vi "Auto_Path Tracking_Security_KBS_TCP.vi"() -> ()   [LabVIEW 2015]
uses:
  <vilib>/Instr/_visa.llb/VISA Configure Serial Port (Instr).vi
  <vilib>/Utility/file.llb/Read Delimited Spreadsheet (DBL).vi
panel:
  in  "M/A":bool=TRUE
  out "bytes written":i32
  out "Tracking_Error(m)":dbl
  in  "SAVE":bool
  out "save state":bool
  out "F9P GPS Data":T1
  out "LidarSteers":T2
  out "ROIs":cluster{bool[]}
  in  "?":enum32{"State", "ETC", "GPS&BATT", "TCP"}(tab)
  in  "stop":bool
  in  "file path (dialog if empty)":path caption="RDDF"
  out "XY Graph":T3(graph)
  in  "Refresh":bool
  in  "Serial Name":refnum<visa-resource-name>="COM1"
  out "ERP_Serial_DATA(RAW)":string
  in  "Vel":u8=4
  out "AEB":bool
  out "Index(near vehicle)":i32
  out "WP_no.":i32
  in  "TCP 수동":bool
  out "x_lat_path":dbl[](array[numeric])
  out "y_long_path":dbl[](array[numeric])
  out "vel. path":dbl[](array[numeric])
  out "Path_Vel_arr":dbl[](array[numeric])
  out "Path_long_arr":dbl[](array[numeric])
  out "Path_lat_arr":dbl[](array[numeric])
  out "ERP_Receive":T4
  out "Steer_CMD(Deg)":dbl
  out "CMD_2_ERP":T5
  in  "COM":refnum<visa-resource-name>="COM12"
  out "Heading_M":dbl
  out "Heading_T":dbl
  out "F9P_Data_GPGGA_Raw":string
  out "TM_Y(long)":dbl format="%-#_10g M"
  out "TM_X(lat)":dbl format="%-#_10g M"
  in  "COM 2":refnum<visa-resource-name>="COM6"
  out "Batt_Volt":dbl
  out "Charge":dbl
  out "Discharge":dbl
  out "SOC":u8
  in  "Speed_CMD":u16
  in  "Gear_CMD":u8
  in  "Steer_CMD":i16
  in  "Brake_CMD":u8
  out "TCP_Lat":u64
  out "TCP_Long":u64
  out "Brake":u8
  out "Go&Stop_feed":u8
  out "Go&Stop_CMD":u8
  out "E-Stop":u8
  out "Robot_State":u8
  out "Robot_Mode":u8
  out "KHP":dbl
  out "IMU_Output":T6
  out "GPS_KHP":u16
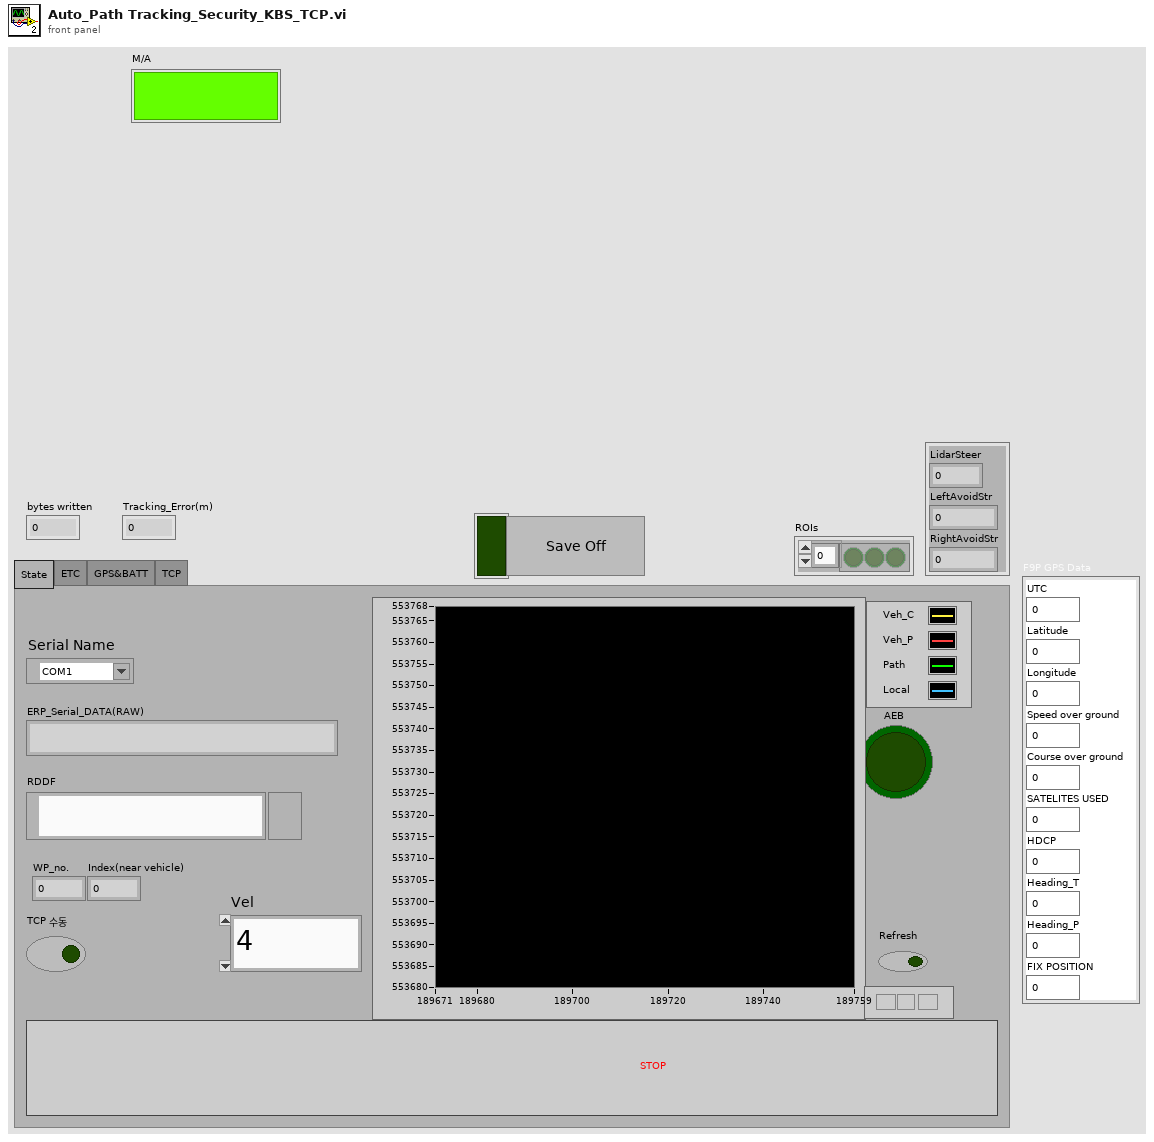
[diagram p1: front panel]
types:
  T1 = cluster{"UTC":dbl, "Latitude":dbl, "Longitude":dbl, "Speed over ground":dbl, "Course over ground":dbl, "SATELITES USED":i32, "HDCP":dbl, "Heading_T":dbl, "Heading_P":dbl, "FIX POSITION":i32}
  T2 = cluster{"LidarSteer":dbl, "LeftAvoidStr":dbl, "RightAvoidStr":dbl}
  T3 = cluster{"y_long_path":dbl[], "x_lat_path":dbl[]}[]
  T4 = cluster{"AorM":u8, "E-Stop":u8, "F_B":u8, "Speed":u16, "Steer":i16, "Brake":u8, "Encoder":u8, "Encoder 2":u8, "Encoder 3":u8, "Encoder 4":u8, "ALIVE":u8, "ETX_0":u8, "ETX_0 2":u8}
  T5 = cluster{"F/B":u8, "Speed":u16, "Steer":i16, "A/M":u8, "Brake":u8}
  T6 = cluster{"Acc_X":dbl, "Acc_Y":dbl, "Acc_Z":dbl, "Gyro_X":dbl, "Gyro_Y":dbl, "Gyro_Z":dbl, "Roll":dbl, "Pitch":dbl, "Yaw":dbl}
  T7 = cluster{"Robot_State_CMD":u8, "Robot_Mode_CMD":u8, "Path_Select":u8, "E-Stop":u8, "F_B":u8, "Speed":u16, "Steer":i16, "Brake":u8}
  T8 = cluster{"BATT_SOC":u8, "Robot_State":u8, "Robot_Mode":u8, "GPS_Lat":u32, "GPS_Long":u32, "Acc_X":i16, "Acc_Y":i16, "Acc_Z":i16, "Gyr_X":i16, "Gyr_Y":i16, "Gyr_Z":i16, "Ang_Roll":i16, "Ang_Pitch":i16, "Ang_Yaw":i16, "GPS_Speed":u16}
  T9 = cluster{"Packet_Size":u16, "Packet_Header":u16, "TCP_Lat":u32, "TCP_Long":u32, "Go&Stop_Feed":u8}
  T10 = enum16{"open", "replace", "create", "open or create", "replace or create", "replace or create with confirmation"}
  T11 = cluster{"S":u8, "T":u8, "X":u8, "AorM":u8, "E-Stop":u8, "F_B":u8, "Speed":u16, "Steer":i16, "Brake":u8, "ALIVE":u8, "ETX_0":u8, "ETX_0 2":u8}
  T12 = cluster{"Path_long_arr":dbl[], "Path_lat_arr":dbl[]}
  T13 = cluster{"Path_long_arr":dbl[], "Path_lat_arr":dbl[]}[]
  T14 = cluster{"UTC":dbl, "Latitude":dbl, "N/S":i8, "Longitude":dbl, "N/S":i8, "FIX POSITION":i32, "SATELITES USED":i32, "HDCP":dbl}
  T15 = cluster{"UTC":dbl, "N/S":i8, "Latitude":dbl, "N/S 2":i8, "Longitude":dbl, "N/S 3":i8, "Speed over ground":dbl, "Course over ground":dbl}
  T16 = cluster{"Heading_T":dbl, "T":i8, "Heading_M":dbl, "M":i8, "G_Speed_Knote":dbl, "N":i8, "G_Speed_KPH":dbl}
  T17 = enum16{"big-endian, network order", "native, host order", "little-endian"}
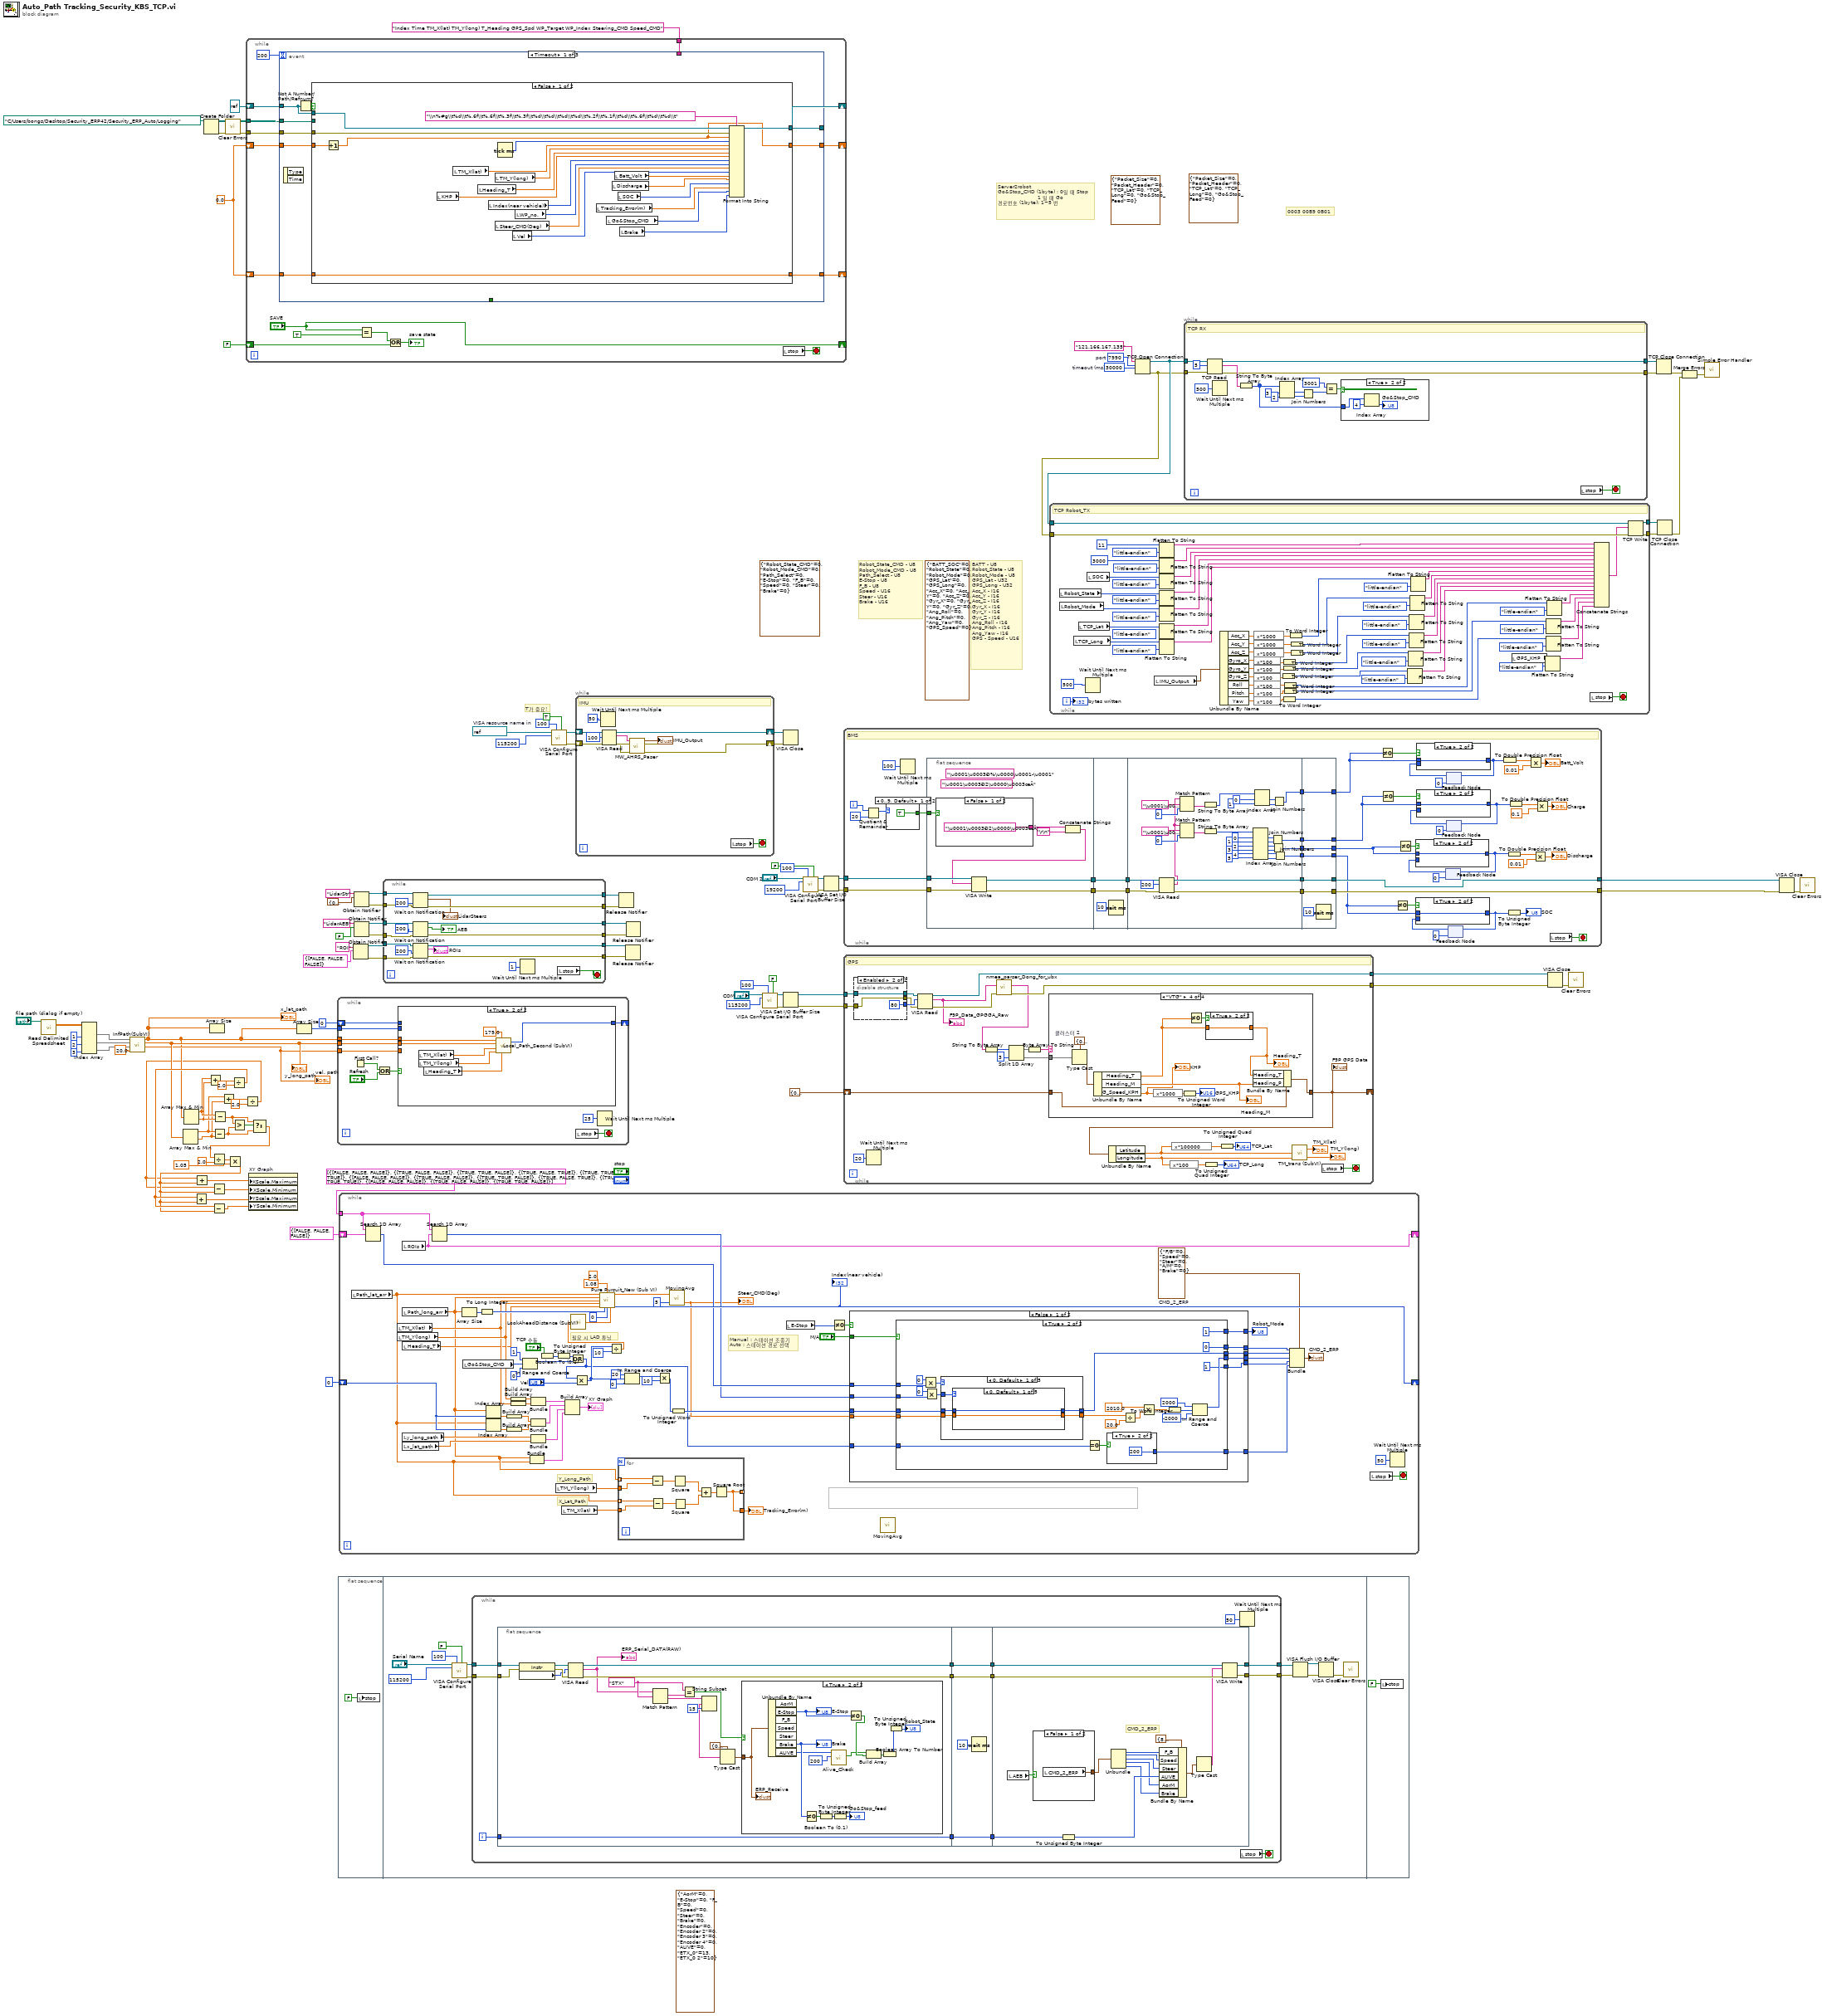
[diagram p0: block diagram]
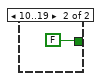
[diagram p7: hidden frame]
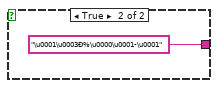
[diagram p8: hidden frame]
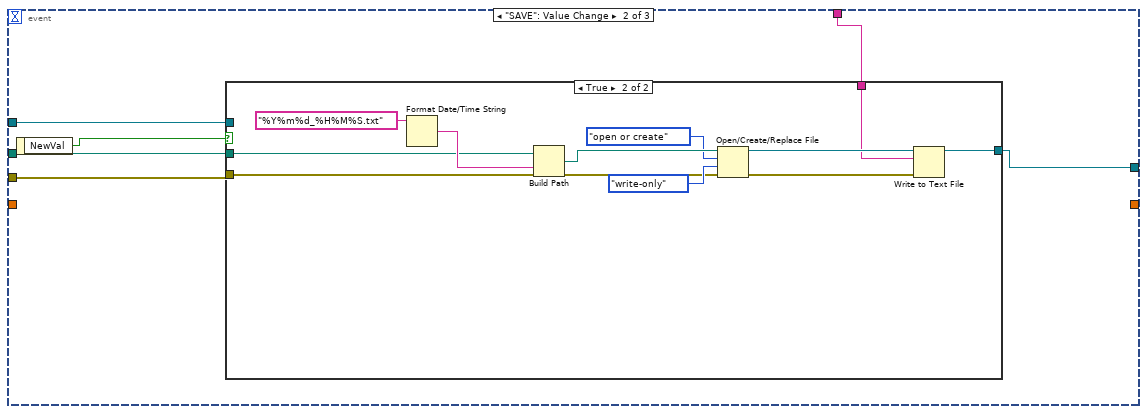
[diagram p10: hidden frame]
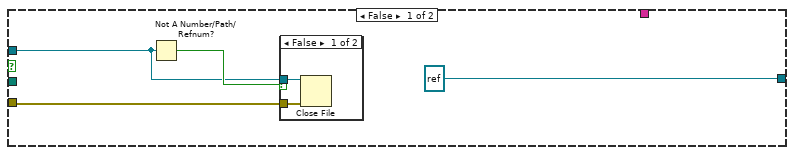
[diagram p11: hidden frame]
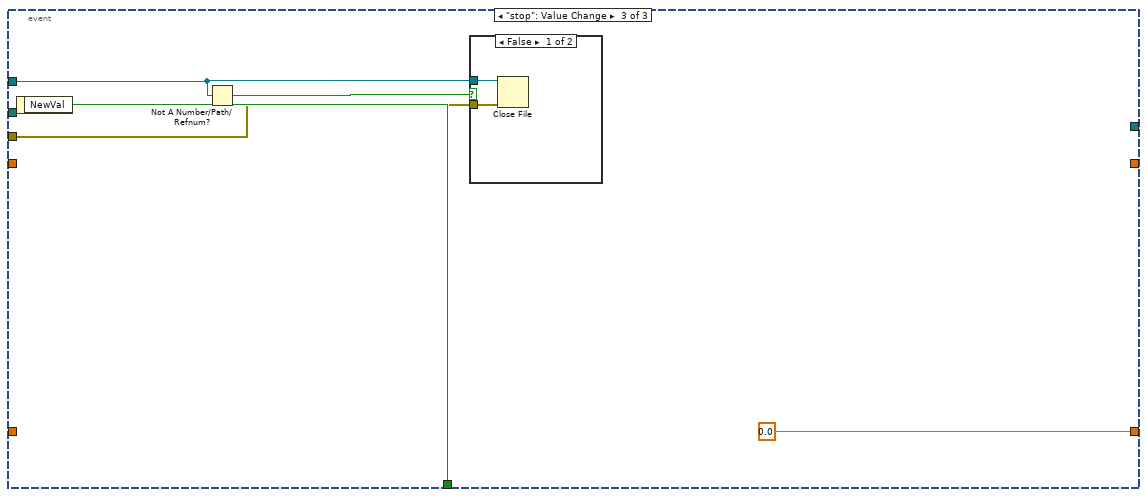
[diagram p13: hidden frame]
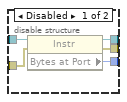
[diagram p15: hidden frame]
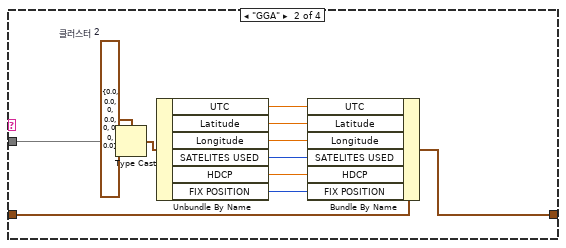
[diagram p17: hidden frame]
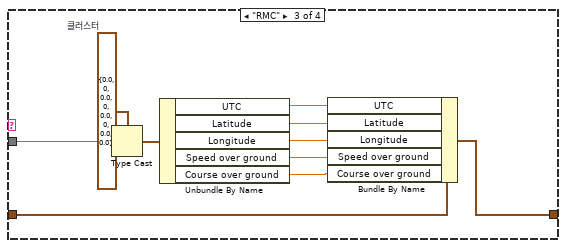
[diagram p18: hidden frame]
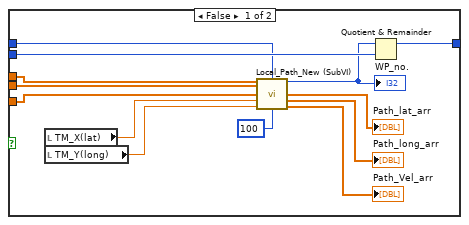
[diagram p20: hidden frame]
diagram:
  (unwired) T4 {"AorM"=0, "E-Stop"=0, "F_B"=0, "Speed"=0, "Steer"=0, "Brake"=0, "Encoder"=0, "Encoder 2"=0, "Encoder 3"=0, "Encoder 4"=0, "ALIVE"=0, "ETX_0"=13, "ETX_0 2"=10}
  (unwired) T7 {"Robot_State_CMD"=0, "Robot_Mode_CMD"=0, "Path_Select"=0, "E-Stop"=0, "F_B"=0, "Speed"=0, "Steer"=0, "Brake"=0} ("Server2Robot")
  (unwired) T8 {"BATT_SOC"=0, "Robot_State"=0, "Robot_Mode"=0, "GPS_Lat"=0, "GPS_Long"=0, "Acc_X"=0, "Acc_Y"=0, "Acc_Z"=0, "Gyr_X"=0, "Gyr_Y"=0, "Gyr_Z"=0, "Ang_Roll"=0, "Ang_Pitch"=0, "Ang_Yaw"=0, "GPS_Speed"=0} ("Robot2Server")
  w2 = u16 7990  # port
  w3 = 30000  # timeout (ms)
  w18 = refnum<visa-resource-name> "COM14"  # VISA resource name in
  (unwired) T9 {"Packet_Size"=0, "Packet_Header"=0, "TCP_Lat"=0, "TCP_Long"=0, "Go&Stop_Feed"=0}
  (unwired) T9 {"Packet_Size"=0, "Packet_Header"=0, "TCP_Lat"=0, "TCP_Long"=0, "Go&Stop_Feed"=0}
  w32 = 0.0 ("Distance(Encoder)")
  # "Robot_State_CMD - U8\nRobot_Mode_CMD - U8\nPath_Select - U8\nE-Stop - U8\nF_B - U8\nSpeed - U16\nSteer - U16\nBrake - U16"
  # "BATT - U8\nRobot_State - U8\nRobot_Mode - U8\nGPS_Lat - U32\nGPS_Long - U32\nAcc_X - I16\nAcc_Y - I16\nAcc_Z - I16\nGyr_X - I16\nGyr_Y - I16\nGyr_Z - I16\nAng_Roll - I16\nAng_Pitch - I16\nAng_Yaw - I16\nGPS - Speed - U16"
  # "T가 중요!"
  # "0003 00B9 0B01"
  # "Server2robot\nGo&Stop_CMD (1byte) : 0일 때 Stop\n                        1 일 때 Go\n경로번호 (1byte): 1~5 번"
  n1 = call-poly <vilib>:"Read Delimited Spreadsheet.vi"("file path (dialog if empty)"="file path (dialog if empty)") -> ("all rows"=w76:dbl[][])  [unwired: 9 in, 5 out]
  n2 = Index Array(array=w76, index (col) #1=1 ("비활성화된 인덱스 (열)"), index (col) #2=2 ("인덱스 (열)"), index (col) #3=3 ("인덱스 (열)")) -> (element #1=w105:dbl[], element #2=w104:dbl[], element #3=w103:dbl[])  [unwired: 3 in]
  n3 = call "InfPath(SubVI).vi"("Mod dist."=20.0, "vel."=w103, "y_long"=w104, "x_lat"=w105) -> ("vel. path"=w78:dbl[], "y_long_path"=w80:dbl[], "x_lat_path"=w77:dbl[])  [unwired: 1 out]
  "x_lat_path" <- w77
  "y_long_path" <- w80
  "vel. path" <- w78
  n4 = Array Max & Min(array=w80) -> (max value=w91:dbl, min value=w90:dbl)  [unwired: 2 out]
  n5 = Array Max & Min(array=w77) -> (max value=w97:dbl, min value=w96:dbl)  [unwired: 2 out]
  n6 = Create Folder(path (use dialog)=path "C:/Users/bongs/Desktop/Security_ERP42/Security_ERP_Auto/Logging") -> (created path=w35:path, error out=w33:errorcluster)  [unwired: 2 in, 1 out]
  n7 = Add(x=w97, y=w96) -> (x+y=w94:dbl)
  n8 = Array Size(array=w77) -> ()  [unwired: 1 out]
  n9 = Subtract(x=w91, y=w90) -> (x-y=w100:dbl)
  n10 = Subtract(x=w97, y=w96) -> (x-y=w101:dbl)
  n11 = Add(x=w91, y=w90) -> (x+y=w93:dbl)
  n12 = call <vilib>:"Clear Errors.vi"("error in (no error)"=w33) -> ("error out"=w34:errorcluster)  [unwired: 5 in, 1 out]
  n13 = Divide(x=w94, y=2.0) -> (x/y=w87:dbl)
  n14 = Greater?(x=w101, y=w100) -> (0:w102:bool)
  n15 = Divide(x=w93, y=2.0) -> (x/y=w74:dbl)
  n16 = while {
    tunnel: w34 -> [w123]
    tunnel: w35 -> [w122]
    shift-right: [w121] -> _
    shift-left: refnum<file> refnum ("refnum out") -> [w120]
    shift-right: [w119] -> _
    shift-left: w32 -> [w118]
    tunnel: "Index Time TM_X(lat) TM_Y(long) T_Heading GPS_Spd WP_Target WP_Index Steering_CMD Speed_CMD" ("포맷 문자열") -> [w117]
    shift-right: [w115] -> _
    shift-left: w32 -> [w116]
    shift-right: ["SAVE"] -> _
    shift-left: FALSE -> [w109]
    stop <- w110 stop-if-true
    n17 = event shown="[0] Timeout" {
      selector: _ -> [_ _ _]
      dyn-events: _ -> [_ _ _]
      timeout: 200 -> [_ _ _]
      tunnel: w123 -> [w131 w162 w183]
      tunnel: w122 -> [w132 w164 _]
      tunnel: [_ _ w186] -> _
      tunnel: [w129 w163 _] -> w121
      tunnel: w120 -> [w130 w160 w184]
      tunnel: [w127 _ 0.0 ("Distance(Encoder)")] -> w119
      tunnel: w118 -> [w128 _ _]
      tunnel: w117 -> [_ w159 _]
      tunnel: w116 -> [w126 _ _]
      tunnel: [w125 _ _] -> w115
      event Timeout {
        n18 = event-data() -> ()  [unwired: 1 in, 2 out]
        n19 = Not A Number/Path/Refnum?(number/path/refnum=w130) -> (NaN/Path/Refnum?=w133:bool)
        n20 = case shown="False" w133 {
          tunnel: w132 -> [_ _]
          tunnel: w131 -> [w155 _]
          tunnel: w130 -> [w154 w158]
          tunnel: [w153 w158] -> w129
          tunnel: w128 -> [w152 w157]
          tunnel: [w152 w157] -> w127
          tunnel: w126 -> [w151 w156]
          tunnel: [w149 w156] -> w125
          frame False {
            n21 = Increment(x=w151) -> (x+1=w149:dbl)
            n22 = local read "KHP"() -> (w144:dbl)
            n23 = local read "TM_X(lat)"() -> (w147:dbl)
            n24 = local read "Heading_T"() -> (w145:dbl)
            n25 = local read "Index(near vehicle)"() -> (w143:i32)
            n26 = local read "TM_Y(long)"() -> (w146:dbl)
            n27 = local read "Steer_CMD(Deg)"() -> (w141:dbl)
            n28 = Tick Count (ms)() -> (millisecond timer value=w148:u32)
            n29 = local read "Vel"() -> (w140:u8)
            n30 = local read "WP_no."() -> (w142:i32)
            n31 = local read "Tracking_Error(m)"() -> (w136:dbl)
            n32 = local read "Go&Stop_CMD"() -> (w135:u8)
            n33 = local read "Discharge"() -> (w138:dbl)
            n34 = local read "Batt_Volt"() -> (w139:dbl)
            n35 = local read "SOC"() -> (w137:u8)
            n36 = local read "Brake"() -> (w134:u8)
            n37 = Format Into String(format string="\\n%#g\\t%d\\t%.6f\\t%.6f\\t%.3f\\t%.3f\\t%d\\t%d\\t%d\\t%d\\t%.2f\\t%.1f\\t%d\\t%.6f\\t%d\\t%d\\t" ("포맷 문자열"), initial string=w154, error in=w155, w149, w148, w147, w146, w145, w144, w143, w142, w141, w140, w139, w138, w137, w136, w135, w134) -> (resulting string=w153:refnum<file>)  [unwired: 1 out]
          }
          frame True {
          }
        }
      }
      event "SAVE": Value Change {
        n38 = event-data() -> ("NewVal"=w161:bool)  [unwired: 1 in]
        n39 = case shown="True" w161 {
          tunnel: w164 -> [_ w179]
          tunnel: [refnum<file> refnum ("refnum out") w173] -> w163
          tunnel: w162 -> [w165 w175]
          tunnel: w160 -> [w167 _]
          tunnel: w159 -> [_ w172]
          frame False {
            n40 = Not A Number/Path/Refnum?(number/path/refnum=w167) -> (NaN/Path/Refnum?=w168:bool)
            n41 = case shown="False" w168 {
              tunnel: w167 -> [w170 _]
              tunnel: w165 -> [w169 _]
              frame False {
                n42 = Close File(refnum=w170, error in=w169) -> ()  [unwired: 2 out]
              }
              frame True {
              }
            }
          }
          frame True {
            n43 = Format Date/Time String(time format string (%c)="%Y%m%d_%H%M%S.txt" ("시간 포맷 문자열 (%c)")) -> (date/time string=w180:string)  [unwired: 2 in]
            n44 = Build Path(base path=w179, name or relative path=w180) -> (appended path=w178:path)
            n45 = Open/Create/Replace File(file path (use dialog)=w178, error in=w175, operation (0:open)=T10."open or create" ("동작(0:open)"), access (0:read/write)=enum16{"read/write", "read-only", "write-only"}."write-only" ("접근(0:읽기/쓰기)")) -> (refnum out=w174:refnum<file>, error out=w171:errorcluster)  [unwired: 2 in, 1 out]
            n46 = Write to Text File(file (use dialog)=w174, text=w172, error in=w171) -> (refnum out=w173:refnum<file>)  [unwired: 1 in, 2 out]
          }
        }
      }
      event "stop": Value Change {
        n47 = event-data() -> ("NewVal"=w186:bool)  [unwired: 1 in]
        n48 = Not A Number/Path/Refnum?(number/path/refnum=w184) -> (NaN/Path/Refnum?=w185:bool)
        n49 = case shown="False" w185 {
          tunnel: w184 -> [w188 _]
          tunnel: w183 -> [w187 _]
          frame False {
            n50 = Close File(refnum=w188, error in=w187) -> ()  [unwired: 2 out]
          }
          frame True {
          }
        }
      }
    }
    n51 = Equal?(x="SAVE", y=TRUE) -> (x = y?=w113:bool)
    n52 = Or(x=w113, y=w109) -> (x .or. y?=→"save state":bool)
    n53 = local read "stop"() -> (w110:bool)
  }
  n54 = Select(t=w101, s=w102, f=w100) -> (s? t:f=w98:dbl)
  n55 = Divide(x=w98, y=2.0) -> (x/y=w89:dbl)
  n56 = Multiply(x=w89, y=1.05) -> (x*y=w86:dbl)
  n57 = Add(x=w87, y=w86) -> (x+y=w84:dbl)
  n58 = Add(x=w74, y=w86) -> (x+y=w82:dbl)
  n59 = Subtract(x=w74, y=w86) -> (x-y=w83:dbl)
  n60 = Subtract(x=w87, y=w86) -> (x-y=w85:dbl)
  n61 = property on="XY Graph" class="XYGraph (strict)"("XScale.Maximum"=w82, "XScale.Minimum"=w83, "YScale.Maximum"=w84, "YScale.Minimum"=w85) -> ()  [unwired: 2 in, 2 out]
  n62 = Array Size(array=w77) -> (size(s)=w79:i32)
  n63 = while {
    tunnel: w77 -> [w198]
    tunnel: w80 -> [w197]
    tunnel: w78 -> [w195]
    tunnel: w79 -> [w194]
    shift-right: [w193] -> _
    shift-left: 0 ("Index0") -> [w196]
    stop <- w199 stop-if-true
    n64 = First Call?() -> (First Call?: T/F=w191:bool)
    n65 = Or(x=w191, y="Refresh") -> (x .or. y?=w192:bool)
    n66 = case shown="True" w192 {
      tunnel: w198 -> [w200 w219]
      tunnel: w197 -> [w202 w218]
      tunnel: w196 -> [w207 _]
      tunnel: w195 -> [w201 _]
      tunnel: w194 -> [w211 _]
      tunnel: [w212 w213] -> w193
      frame False {
        n67 = local read "TM_X(lat)"() -> (w210:dbl)
        n68 = local read "TM_Y(long)"() -> (w209:dbl)
        n69 = call "Local_Path_New (SubVI).vi"("x_lat_arr"=w200, "WP no_pre"=w207, "y_long_arr"=w202, "vel_arr"=w201, "x_lat_c"=w210, "y_long_c"=w209, "# of pnt"=100) -> ("INDEX(Near Point)"=w203:i32, "Lat(Local)"=→"Path_lat_arr":dbl[], "Long(Local)"=→"Path_long_arr":dbl[], "Vel(Local)"=→"Path_Vel_arr":dbl[])  [unwired: 5 in]
        "WP_no." <- w203
        n70 = Quotient & Remainder(x=w203, y=w211) -> (x-y*floor(x/y)=w212:i32)  [unwired: 1 out]
      }
      frame True {
        n71 = local read "TM_X(lat)"() -> (w217:dbl)
        n72 = local read "TM_Y(long)"() -> (w216:dbl)
        n73 = local read "Heading_T"() -> (w215:dbl)
        n74 = call "Local_Path_Second (SubVI).vi"("heading_deg"=w215, "heading_limit"=179.0, "y_long"=w216, "x_lat"=w217, "Y_long_path"=w218, "X_lat_path"=w219) -> ("Index(near vehicle)"=w213:i32)  [unwired: 1 out]
      }
    }
    n75 = local read "stop"() -> (w199:bool)
    n76 = Wait Until Next ms Multiple(millisecond multiple=u32 25) -> ()  [unwired: 1 out]
  }
  n77 = flat-sequence {
    frame #0 {
      n78 = local write "stop"(FALSE ("STop")) -> ()
    }
    frame #1 {
      n79 = call-poly "VISA Configure Serial Port"("VISA resource name"="Serial Name", "timeout (10sec)"=u32 100, "Enable Termination\nChar (T)"=FALSE ("Enable Termination\nChar (T)"), "baud rate (9600)"=u32 115200) -> ("VISA resource name out"=w223:refnum<visa-resource-name>, "error out"=w222:errorcluster)  [unwired: 10 in]
      n80 = while {
        tunnel: w223 -> [w243]
        tunnel: w222 -> [w242]
        tunnel: [w240] -> w225
        tunnel: [w239] -> w224
        i -> [w241]
        stop <- w232 stop-if-true
        n81 = flat-sequence {
          tunnel: w243 -> [w261]
          tunnel: w242 -> [w260]
          tunnel: [w259] -> w238
          tunnel: [w258] -> w236
          tunnel: w241 -> [w257]
          tunnel: [w257] -> w234
          tunnel: w238 -> [w278]
          tunnel: [w278] -> w237
          tunnel: w236 -> [w277]
          tunnel: [w277] -> w235
          tunnel: w234 -> [w276]
          tunnel: [w276] -> w233
          tunnel: w237 -> [w292]
          tunnel: w235 -> [w291]
          tunnel: w233 -> [w289]
          tunnel: [w288] -> w240
          tunnel: [w287] -> w239
          frame #0 {
            w251 = "STX" ("검색 문자열/문자 (-)")
            n82 = property class="Instr"(reference=w261, error in=w260) -> (reference out=w254:refnum<visa-resource-name>, error out=w256:errorcluster, "Serial Settings:Number of Bytes at Serial Port"=w255:u32)
            n83 = VISA Read(VISA resource name=w254, byte count=w255, error in (no error)=w256) -> (VISA resource name out=w259:refnum<visa-resource-name>, read buffer=w249:string, error out=w258:errorcluster)  [unwired: 1 out]
            "ERP_Serial_DATA(RAW)" <- w249
            n84 = Match Pattern(string=w249, regular expression=w251) -> (match substring=w250:string, after substring=w253:string)  [unwired: 1 in, 2 out]
            n85 = Equal?(x=w251, y=w250) -> (x = y?=w248:bool)
            n86 = String Subset(string=w253, length (rest)=15 ("길이(나머지)")) -> (substring=w247:string)  [unwired: 1 in]
            n87 = Type Cast(type=T4 {"AorM"=0, "E-Stop"=0, "F_B"=0, "Speed"=0, "Steer"=0, "Brake"=0, "Encoder"=0, "Encoder 2"=0, "Encoder 3"=0, "Encoder 4"=0, "ALIVE"=0, "ETX_0"=13, "ETX_0 2"=10}, x=w247) -> (*(type *) &x=w245:T4)
            n88 = case shown="True" w248 {
              tunnel: w245 -> [_ w270]
              frame False {
              }
              frame True {
                n89 = Unbundle By Name(w270) -> ("E-Stop"=w267:u8, "Brake"=w274:u8, "ALIVE"=w269:u8)  [unwired: 4 out]
                "Brake" <- w274
                "E-Stop" <- w267
                n90 = Not Equal To 0?(x=w274) -> (x != 0?=w273:bool)
                n91 = Boolean To (0,1)(Boolean=w273) -> (0, 1=w272:i16)
                n92 = call "Alive_Check.vi"("Timeout_msec"=u32 200, "Alv_cnt"=w269) -> ("Timeout"=w262:bool)  [unwired: 8 in, 1 out]
                n93 = To Unsigned Byte Integer(number=w272) -> (unsigned 8bit integer=→"Go&Stop_feed":u8)
                n94 = Not Equal To 0?(x=w267) -> (x != 0?=w263:bool)
                n95 = Build Array(w262, w263) -> (w266:bool[])
                n96 = Boolean Array To Number(Boolean array=w266) -> (number=w265:u32)
                n97 = To Unsigned Byte Integer(number=w265) -> (unsigned 8bit integer=→"Robot_State":u8)
                "ERP_Receive" <- w270
              }
            }
          }
          frame #1 {
            n98 = Wait (ms)(milliseconds to wait=u32 10 ("대기 시간(ms)")) -> ()  [unwired: 1 out]
          }
          frame #2 {
            # "CMD_2_ERP"
            n99 = local read "AEB"() -> (w280:bool)
            n100 = case shown="False" w280 {
              tunnel: [w295 w296] -> w281
              frame False {
                n101 = local read "CMD_2_ERP"() -> (w295:T5)
              }
              frame True {
                w296 = T5 {"F/B"=0, "Speed"=0, "Steer"=0, "A/M"=1, "Brake"=200}  # CMD_2_ERP
              }
            }
            n102 = To Unsigned Byte Integer(number=w289) -> (unsigned 8bit integer=w294:u8)
            n103 = Unbundle(w281) -> ("F/B"=w286:u8, "Speed"=w285:u16, "Steer"=w284:i16, "A/M"=w282:u8, "Brake"=w279:u8)
            n104 = Bundle By Name(cluster=T11 {"S"=83, "T"=84, "X"=88, "AorM"=0, "E-Stop"=0, "F_B"=0, "Speed"=0, "Steer"=0, "Brake"=0, "ALIVE"=0, "ETX_0"=13, "ETX_0 2"=10}, "F_B"=w286, "Speed"=w285, "Steer"=w284, "ALIVE"=w294, "AorM"=w282, "Brake"=w279) -> (w293:T11)
            n105 = Type Cast(x=w293) -> (*(type *) &x=w290:string)  [unwired: 1 in]
            n106 = VISA Write(VISA resource name=w292, write buffer=w290, error in (no error)=w291) -> (VISA resource name out=w288:refnum<visa-resource-name>, error out=w287:errorcluster)  [unwired: 1 out]
          }
        }
        n107 = Wait Until Next ms Multiple(millisecond multiple=u32 50 ("ms 배수")) -> ()  [unwired: 1 out]
        n108 = local read "stop"() -> (w232:bool)
      }
      n109 = VISA Flush I/O Buffer(VISA resource name=w225, error in (no error)=w224) -> (VISA resource name out=w226:refnum<visa-resource-name>, error out=w227:errorcluster)  [unwired: 1 in]
      n110 = VISA Close(VISA resource name=w226, error in (no error)=w227) -> (error out=w221:errorcluster)
      n111 = call <vilib>:"Clear Errors.vi"("error in (no error)"=w221) -> ()  [unwired: 5 in, 2 out]
    }
    frame #2 {
      n112 = local write "stop"(FALSE ("STop")) -> ()
    }
  }
  n113 = while {
    shift-right: [w351] -> _
    shift-left: 0 -> [w346]
    shift-right: [w330] -> _
    shift-left: cluster{bool[]} {[FALSE, FALSE, FALSE]} -> [w333]
    tunnel: cluster{bool[]}[] [{[FALSE, FALSE, FALSE]}, {[TRUE, FALSE, FALSE]}, {[TRUE, TRUE, FALSE]}, {[TRUE, FALSE, TRUE]}, {[TRUE, TRUE, TRUE]}, {[FALSE, FALSE, FALSE]}, {[TRUE, FALSE, FALSE]}, {[TRUE, TRUE, FALSE]}, {[TRUE, FALSE, TRUE]}, {[TRUE, TRUE, TRUE]}, {[FALSE, FALSE, FALSE]}, {[TRUE, FALSE, FALSE]}, {[TRUE, TRUE, FALSE]}] -> [w334]
    stop <- w355 stop-if-true
    w317 = T5 {"F/B"=0, "Speed"=0, "Steer"=0, "A/M"=0, "Brake"=0}  # CMD_2_ERP
    (unwired) 2.0 ("L")
    # "Manual : 스테이션 조종기\nAuto : 스테이션 경로 선택"
    # "X_Lat_Path"
    # "Y_Long_Path"
    # "필요 시 LAD 튜닝"
    n114 = local read "Path_lat_arr"() -> (w309:dbl[])
    n115 = Search 1D Array(1D array=w334, element=w333) -> (index of element=w332:i32)  [unwired: 1 in]
    n116 = local read "TM_X(lat)"() -> (w347:dbl)
    n117 = local read "TM_Y(long)"() -> (w348:dbl)
    n118 = local read "y_long_path"() -> (w323:dbl[])
    n119 = local read "x_lat_path"() -> (w322:dbl[])
    n120 = local read "ROIs"() -> (w330:cluster{bool[]})
    n121 = local read "Path_long_arr"() -> (w310:dbl[])
    n122 = local read "Heading_T"() -> (w342:dbl)
    n123 = Search 1D Array(1D array=w334, element=w330) -> (index of element=w331:i32)  [unwired: 1 in]
    n124 = Array Size(array=w310) -> (size(s)=w352:i32)
    n125 = local read "Go&Stop_CMD"() -> (w311:u8)
    n126 = To Long Integer(number=w352) -> (32bit integer=w350:i32)
    n127 = Index Array(array=w310, index=w346) -> (element=w359:dbl)
    n128 = Index Array(array=w309, index=w346) -> (element=w358:dbl)
    n129 = Build Array(w359) -> (w357:dbl[])
    n130 = Build Array(w358) -> (w356:dbl[])
    n131 = Build Array(w348) -> (w361:dbl[])
    n132 = Build Array(w347) -> (w360:dbl[])
    n133 = In Range and Coerce(upper limit=u8 1, x=w311, lower limit=u8 0) -> (coerced(x)=w308:u8)  [unwired: 1 out]
    n134 = Bundle("Path_long_arr"=w310, "Path_lat_arr"=w309) -> (w338:T12)  [unwired: 1 in]
    n135 = Bundle(w361, w360) -> (w344:cluster{dbl[], dbl[]})  [unwired: 1 in]
    n136 = Bundle(w357, w356) -> (w343:cluster{dbl[], dbl[]})  [unwired: 1 in]
    n137 = Bundle("y_long_path"=w323, "x_lat_path"=w322) -> (w345:cluster{"y_long_path":dbl[], "x_lat_path":dbl[]})  [unwired: 1 in]
    n138 = Boolean To (0,1)(Boolean="TCP 수동") -> (0, 1=w307:i16)
    n139 = local read "TM_Y(long)"() -> (w320:dbl)
    n140 = To Unsigned Byte Integer(number=w307) -> (unsigned 8bit integer=w305:u8)
    n141 = local read "TM_X(lat)"() -> (w321:dbl)
    n142 = Build Array(w344, w343, w345, w338) -> (→"XY Graph":T13)
    n143 = Or(x=w305, y=w308) -> (x .or. y?=w304:u8)
    n144 = Multiply(x=w304, y="Vel") -> (x*y=w312:u8)
    n145 = Divide(x=w312, y=u8 10) -> (x/y=w339:dbl)
    n146 = call "LookAheadDistance (SubVI).vi"("velocity(kph)"=w339) -> ("ld(m)"=w341:dbl)
    n147 = call "Pure Pursuit_New (Sub VI).vi"("x_lat_path"=w309, "L"=1.08, "y_long_path"=w310, "X_Current"=w347, "Y_Current"=w348, "Heading_Current"=w342, "#pnt"=w350, "WP no_pre"=0, "LAD"=w341) -> ("Steer_CMD(Deg)"=w302:dbl, "Index(near vehicle)"=w351:i32)  [unwired: 5 in]
    "Index(near vehicle)" <- w351
    n148 = for {
      tunnel: w310 -> [w374] mode=indexing
      tunnel: w309 -> [w372] mode=indexing
      tunnel: w321 -> [w371]
      tunnel: w320 -> [w373]
      tunnel: [w365] -> _ mode=indexing
      tunnel: [w365] -> w319
      n149 = Subtract(x=w374, y=w373) -> (x-y=w370:dbl)
      n150 = Subtract(x=w372, y=w371) -> (x-y=w369:dbl)
      n151 = Square(x=w370) -> (x^2=w368:dbl)
      n152 = Square(x=w369) -> (x^2=w367:dbl)
      n153 = Add(x=w368, y=w367) -> (x+y=w366:dbl)
      n154 = Square Root(x=w366) -> (sqrt(x)=w365:dbl)
    }
    "Tracking_Error(m)" <- w319
    n155 = In Range and Coerce(upper limit=u8 20 ("상위 리미트"), x=w312, lower limit=u8 0 ("하위 리미트")) -> (coerced(x)=w327:u8)  [unwired: 1 out]
    n156 = Multiply(x=w327, y=u8 10) -> (x*y=w325:u8)
    n157 = call "MovingAvg.vi"("입력"=w302, "이동평균을 구할 자료의 개수"=u16 5) -> ("이동평균"=w301:dbl)  [unwired: 2 out]
    "Steer_CMD(Deg)" <- w301
    n158 = To Unsigned Word Integer(number=w325) -> (unsigned 16bit integer=w336:u16)
    n159 = local read "E-Stop"() -> (w299:u8)
    n160 = Not Equal To 0?(x=w299) -> (x != 0?=w335:bool)
    n161 = case shown="False" w335 {
      tunnel: [w378 w518] -> w364
      tunnel: [w384 w518] -> w363
      tunnel: [w383 w518] -> w362
      tunnel: [w377 w518] -> w337
      tunnel: w332 -> [w382 _]
      tunnel: w331 -> [w381 _]
      tunnel: w301 -> [w386 _]
      tunnel: w336 -> [w385 _]
      tunnel: [w380 u8 200] -> w318
      tunnel: w304 -> [w379 _]
      tunnel: "M/A" -> [w376 _]
      tunnel: [w375 w518] -> w298
      frame False {
        n162 = case shown="True" w376 {
          tunnel: w386 -> [_ w425]
          tunnel: w385 -> [_ w424]
          tunnel: [w397 w423] -> w384
          tunnel: [w392 w414] -> w383
          tunnel: w382 -> [_ w413]
          tunnel: w381 -> [_ w409]
          tunnel: [w387 w407] -> w380
          tunnel: w379 -> [_ w406]
          tunnel: ["Gear_CMD" u8 0] -> w378
          tunnel: [u8 1 u8 1] -> w377
          tunnel: [u8 0 u8 1] -> w375
          frame False {
            n163 = In Range and Coerce(upper limit=i16 2000, x="Steer_CMD", lower limit=i16 -2000) -> (coerced(x)=w392:i16)  [unwired: 1 out]
            n164 = In Range and Coerce(upper limit=u16 10, x="Speed_CMD", lower limit=u16 0) -> (coerced(x)=w397:u16)  [unwired: 1 out]
            n165 = In Range and Coerce(upper limit=u8 200, x="Brake_CMD", lower limit=u8 0) -> (coerced(x)=w387:u8)  [unwired: 1 out]
          }
          frame True {
            n166 = Multiply(x=0, y=w413) -> (x*y=w411:i32)
            n167 = Multiply(x=0, y=w409) -> (x*y=w408:i32)
            n168 = case shown="0, Default" w411 {
              tunnel: w425 -> [w430 w448 w466 w484 w502]
              tunnel: [w431 w449 w467 w485 w503] -> w415
              tunnel: w408 -> [w432 w450 w468 w486 w504]
              tunnel: [w429 w447 w465 w483 w501] -> w423
              tunnel: w424 -> [w428 w446 w464 w482 w500]
              frame 0, Default {
                n169 = case shown="0, Default" w432 {
                  tunnel: [w434 w436 w438 w441 w444] -> w431
                  tunnel: w430 -> [w434 w436 _ _ _]
                  tunnel: [w433 w435 w437 w440 w443] -> w429
                  tunnel: w428 -> [w433 w435 w437 w440 w443]
                  frame 0, Default {
                  }
                  frame 1 {
                  }
                  frame 2 {
                    n170 = local read "LidarSteers"() -> (w439:T2)
                    n171 = Unbundle By Name(w439) -> ("LeftAvoidStr"=w438:dbl)
                  }
                  frame 3 {
                    n172 = local read "LidarSteers"() -> (w442:T2)
                    n173 = Unbundle By Name(w442) -> ("RightAvoidStr"=w441:dbl)
                  }
                  frame 4 {
                    n174 = local read "LidarSteers"() -> (w445:T2)
                    n175 = Unbundle By Name(w445) -> ("LidarSteer"=w444:dbl)
                  }
                }
              }
              frame 1 {
                n176 = case shown="0, Default" w450 {
                  tunnel: [w452 w454 w456 w459 w462] -> w449
                  tunnel: w448 -> [w452 w454 _ _ _]
                  tunnel: [w451 w453 w455 w458 w461] -> w447
                  tunnel: w446 -> [w451 w453 w455 w458 w461]
                  frame 0, Default {
                  }
                  frame 1 {
                  }
                  frame 2 {
                    n177 = local read "LidarSteers"() -> (w457:T2)
                    n178 = Unbundle By Name(w457) -> ("LeftAvoidStr"=w456:dbl)
                  }
                  frame 3 {
                    n179 = local read "LidarSteers"() -> (w460:T2)
                    n180 = Unbundle By Name(w460) -> ("RightAvoidStr"=w459:dbl)
                  }
                  frame 4 {
                    n181 = local read "LidarSteers"() -> (w463:T2)
                    n182 = Unbundle By Name(w463) -> ("LidarSteer"=w462:dbl)
                  }
                }
              }
              frame 2 {
                n183 = case shown="1" w468 {
                  tunnel: [w470 w472 w474 w477 w480] -> w467
                  tunnel: w466 -> [w470 w472 _ _ _]
                  tunnel: [w469 w471 w473 w476 w479] -> w465
                  tunnel: w464 -> [w469 w471 w473 w476 w479]
                  frame 0, Default {
                  }
                  frame 1 {
                  }
                  frame 2 {
                    n184 = local read "LidarSteers"() -> (w475:T2)
                    n185 = Unbundle By Name(w475) -> ("LeftAvoidStr"=w474:dbl)
                  }
                  frame 3 {
                    n186 = local read "LidarSteers"() -> (w478:T2)
                    n187 = Unbundle By Name(w478) -> ("RightAvoidStr"=w477:dbl)
                  }
                  frame 4 {
                    n188 = local read "LidarSteers"() -> (w481:T2)
                    n189 = Unbundle By Name(w481) -> ("LidarSteer"=w480:dbl)
                  }
                }
              }
              frame 3 {
                n190 = case shown="0, Default" w486 {
                  tunnel: [w488 w490 w492 w495 w498] -> w485
                  tunnel: w484 -> [w488 w490 _ _ _]
                  tunnel: [w487 w489 w491 w494 w497] -> w483
                  tunnel: w482 -> [w487 w489 w491 w494 w497]
                  frame 0, Default {
                  }
                  frame 1 {
                  }
                  frame 2 {
                    n191 = local read "LidarSteers"() -> (w493:T2)
                    n192 = Unbundle By Name(w493) -> ("LeftAvoidStr"=w492:dbl)
                  }
                  frame 3 {
                    n193 = local read "LidarSteers"() -> (w496:T2)
                    n194 = Unbundle By Name(w496) -> ("RightAvoidStr"=w495:dbl)
                  }
                  frame 4 {
                    n195 = local read "LidarSteers"() -> (w499:T2)
                    n196 = Unbundle By Name(w499) -> ("LidarSteer"=w498:dbl)
                  }
                }
              }
              frame 4 {
                n197 = case shown="0, Default" w504 {
                  tunnel: [w506 w508 w510 w513 w516] -> w503
                  tunnel: w502 -> [w506 w508 _ _ _]
                  tunnel: [w505 w507 w509 w512 w515] -> w501
                  tunnel: w500 -> [w505 w507 w509 w512 w515]
                  frame 0, Default {
                  }
                  frame 1 {
                  }
                  frame 2 {
                    n198 = local read "LidarSteers"() -> (w511:T2)
                    n199 = Unbundle By Name(w511) -> ("LeftAvoidStr"=w510:dbl)
                  }
                  frame 3 {
                    n200 = local read "LidarSteers"() -> (w514:T2)
                    n201 = Unbundle By Name(w514) -> ("RightAvoidStr"=w513:dbl)
                  }
                  frame 4 {
                    n202 = local read "LidarSteers"() -> (w517:T2)
                    n203 = Unbundle By Name(w517) -> ("LidarSteer"=w516:dbl)
                  }
                }
              }
            }
            n204 = Equal To 0?(x=w406) -> (x = 0?=w405:bool)
            n205 = case shown="True" w405 {
              tunnel: [u8 0 u8 200] -> w407
              frame False {
              }
              frame True {
              }
            }
            n206 = Divide(x=w415, y=20.0) -> (x/y=w421:dbl)
            n207 = Multiply(x=2010.0, y=w421) -> (x*y=w420:dbl)
            n208 = To Word Integer(number=w420) -> (16bit integer=w422:i16)
            n209 = In Range and Coerce(upper limit=i16 2000 ("상위 리미트"), x=w422, lower limit=i16 -2000 ("하위 리미트")) -> (coerced(x)=w414:i16)  [unwired: 1 out]
          }
        }
      }
      frame True {
        w518 = u8 0
      }
    }
    "Robot_Mode" <- w298
    n210 = call "MovingAvg.vi"() -> ()  [unwired: 2 in, 3 out]
    n211 = Bundle(cluster=w317, "F/B"=w364, "Speed"=w363, "Steer"=w362, "A/M"=w337, "Brake"=w318) -> (→"CMD_2_ERP":T5)
    n212 = local read "stop"() -> (w355:bool)
    n213 = Wait Until Next ms Multiple(millisecond multiple=u32 50 ("ms 배수")) -> ()  [unwired: 1 out]
  }
  n214 = Obtain Notifier(name (unnamed)="ROI" ("이름(이름없음)"), notification data type=cluster{bool[]} {[FALSE, FALSE, FALSE]}) -> (notifier out=w58:refnum<notifier>, error out=w57:errorcluster)  [unwired: 2 in, 1 out]
  n215 = Obtain Notifier(name (unnamed)="LidarStr" ("이름(이름없음)"), notification data type=T2 {"LidarSteer"=0.0, "LeftAvoidStr"=0.0, "RightAvoidStr"=0.0}) -> (notifier out=w71:refnum<notifier>, error out=w69:errorcluster)  [unwired: 2 in, 1 out]
  n216 = Obtain Notifier(name (unnamed)="LidarAEB" ("이름(이름없음)"), notification data type=FALSE) -> (notifier out=w65:refnum<notifier>, error out=w62:errorcluster)  [unwired: 2 in, 1 out]
  n217 = while {
    tunnel: w71 -> [w537]
    tunnel: [w536] -> w70
    tunnel: w69 -> [w535]
    tunnel: [w534] -> w68
    tunnel: w65 -> [w533]
    tunnel: [w532] -> w64
    tunnel: w62 -> [w531]
    tunnel: [w529] -> w61
    tunnel: w58 -> [w526]
    tunnel: w57 -> [w525]
    tunnel: [w523] -> w56
    tunnel: [w522] -> w55
    stop <- w539 stop-if-true
    n218 = Wait on Notification(notifier=w537, timeout in ms (-1)=200 ("타임아웃(ms) (-1)"), error in (no error)=w535) -> (notifier out=w536:refnum<notifier>, notification=→"LidarSteers":T2, error out=w534:errorcluster)  [unwired: 1 in, 1 out]
    n219 = Wait on Notification(notifier=w533, timeout in ms (-1)=200 ("타임아웃(ms) (-1)"), error in (no error)=w531) -> (notifier out=w532:refnum<notifier>, notification=→"AEB":bool, error out=w529:errorcluster)  [unwired: 1 in, 1 out]
    n220 = Wait on Notification(notifier=w526, timeout in ms (-1)=200 ("타임아웃(ms) (-1)"), error in (no error)=w525) -> (notifier out=w523:refnum<notifier>, notification=→"ROIs":cluster{bool[]}, error out=w522:errorcluster)  [unwired: 1 in, 1 out]
    n221 = Wait Until Next ms Multiple(millisecond multiple=u32 1) -> ()  [unwired: 1 out]
    n222 = local read "stop"() -> (w539:bool)
  }
  n223 = call-poly "VISA Configure Serial Port"("VISA resource name"=w18, "timeout (10sec)"=u32 100, "Enable Termination\nChar (T)"=TRUE, "baud rate (9600)"=u32 115200) -> ("VISA resource name out"=w17:refnum<visa-resource-name>, "error out"=w16:errorcluster)  [unwired: 10 in]
  n224 = while {
    shift-right: [w549] -> w13
    shift-left: w17 -> [w545]
    shift-right: [w542] -> w12
    shift-left: w16 -> [w544]
    stop <- w541 stop-if-true
    # "IMU"
    n225 = Wait Until Next ms Multiple(millisecond multiple=u32 50) -> ()  [unwired: 1 out]
    n226 = VISA Read(VISA resource name=w545, byte count=u32 100, error in (no error)=w544) -> (VISA resource name out=w549:refnum<visa-resource-name>, read buffer=w547:string, error out=w548:errorcluster)  [unwired: 1 out]
    n227 = call "MW_AHRS_Paser.vi"("error"=w548, "String In"=w547) -> ("error IO"=w542:errorcluster, "Output"=→"IMU_Output":T6)  [unwired: 4 in]
    n228 = local read "stop"() -> (w541:bool)
  }
  n229 = Release Notifier(notifier=w70, error in (no error)=w68) -> ()  [unwired: 1 in, 3 out]
  n230 = Release Notifier(notifier=w56, error in (no error)=w55) -> ()  [unwired: 1 in, 3 out]
  n231 = Release Notifier(notifier=w64, error in (no error)=w61) -> ()  [unwired: 1 in, 3 out]
  n232 = call-poly "VISA Configure Serial Port"("VISA resource name"="COM", "timeout (10sec)"=u32 100, "Enable Termination\nChar (T)"=FALSE ("Enable Termination\nChar (T)"), "baud rate (9600)"=u32 115200 ("baud rate")) -> ("VISA resource name out"=w48:refnum<visa-resource-name>, "error out"=w47:errorcluster)  [unwired: 10 in]
  n233 = VISA Close(VISA resource name=w13, error in (no error)=w12) -> ()  [unwired: 1 out]
  n234 = VISA Set I/O Buffer Size(VISA resource name=w48, error in (no error)=w47) -> (VISA resource name out=w43:refnum<visa-resource-name>, error out=w42:errorcluster)  [unwired: 2 in]
  n235 = call-poly "VISA Configure Serial Port"("VISA resource name"="COM 2", "timeout (10sec)"=u32 100, "Enable Termination\nChar (T)"=FALSE ("Enable Termination\nChar (T)"), "baud rate (9600)"=u32 19200 ("baud rate")) -> ("VISA resource name out"=w28:refnum<visa-resource-name>, "error out"=w27:errorcluster)  [unwired: 10 in]
  n236 = VISA Set I/O Buffer Size(VISA resource name=w28, error in (no error)=w27) -> (VISA resource name out=w24:refnum<visa-resource-name>, error out=w23:errorcluster)  [unwired: 2 in]
  n237 = while {
    shift-right: [w568] -> _
    shift-left: T1 {"UTC"=0.0, "Latitude"=0.0, "Longitude"=0.0, "Speed over ground"=0.0, "Course over ground"=0.0, "SATELITES USED"=0, "HDCP"=0.0, "Heading_T"=0.0, "Heading_P"=0.0, "FIX POSITION"=0} ("Garmin GPS Data") -> [w576]
    tunnel: w43 -> [w560]
    tunnel: w42 -> [w558]
    tunnel: [w569] -> w46
    tunnel: [w575] -> w45
    stop <- w555 stop-if-true
    # "GPS"
    n238 = disable-structure shown="Enabled" {
      disable-tunnel: [w581 u32 80 ("Bytes at Port")] -> w561
      disable-tunnel: w560 -> [w580 w583]
      disable-tunnel: [w579 w583] -> w559
      disable-tunnel: w558 -> [w578 w582]
      disable-tunnel: [w577 w582] -> w557
      frame Disabled {
        n239 = property class="Instr"(reference=w580, error in=w578) -> (reference out=w579:refnum<visa-resource-name>, error out=w577:errorcluster, "Bytes at Port"=w581:u32)
      }
      frame Enabled {
      }
    }
    n240 = Wait Until Next ms Multiple(millisecond multiple=u32 20 ("타임아웃(ms) (-1)")) -> ()  [unwired: 1 out]
    n241 = VISA Read(VISA resource name=w559, byte count=w561, error in (no error)=w557) -> (VISA resource name out=w569:refnum<visa-resource-name>, read buffer=w570:string, error out=w574:errorcluster)  [unwired: 1 out]
    "F9P_Data_GPGGA_Raw" <- w570
    n242 = call "nmea_parser_Dong_for_ubx.vi"("error in"=w574, "INPUT"=w570) -> ("error out"=w575:errorcluster, "output"=w562:string)  [unwired: 8 in]
    n243 = String To Byte Array(string=w562) -> (unsigned byte array=w566:u8[])
    n244 = Split 1D Array(array=w566, index=3) -> (first subarray=w565:u8[], second subarray=w564:u8[])
    n245 = Byte Array To String(unsigned byte array=w565) -> (string=w563:string)
    n246 = case shown="\"VTG\"" w563 {
      tunnel: w564 -> [_ w596 w604 w618]
      tunnel: w576 -> [w585 w592 w603 w614]
      tunnel: [w585 w591 w602 w615] -> w568
      frame Default {
      }
      frame "GGA" {
        w594 = T14 {"UTC"=0.0, "Latitude"=0.0, "N/S"=0, "Longitude"=0.0, "N/S"=0, "FIX POSITION"=0, "SATELITES USED"=0, "HDCP"=0.0}  # 클러스터 2
        n247 = Type Cast(type=w594, x=w596) -> (*(type *) &x=w595:T14)
        n248 = Unbundle By Name(w595) -> ("UTC"=w593:dbl, "Latitude"=w590:dbl, "Longitude"=w589:dbl, "SATELITES USED"=w588:i32, "HDCP"=w587:dbl, "FIX POSITION"=w586:i32)
        n249 = Bundle By Name(cluster=w592, "UTC"=w593, "Latitude"=w590, "Longitude"=w589, "SATELITES USED"=w588, "HDCP"=w587, "FIX POSITION"=w586) -> (w591:T1)
      }
      frame "RMC" {
        w606 = T15 {"UTC"=0.0, "N/S"=0, "Latitude"=0.0, "N/S 2"=0, "Longitude"=0.0, "N/S 3"=0, "Speed over ground"=0.0, "Course over ground"=0.0}  # 클러스터
        n250 = Type Cast(type=w606, x=w604) -> (*(type *) &x=w605:T15)
        n251 = Unbundle By Name(w605) -> ("UTC"=w601:dbl, "Latitude"=w600:dbl, "Longitude"=w599:dbl, "Speed over ground"=w598:dbl, "Course over ground"=w597:dbl)
        n252 = Bundle By Name(cluster=w603, "UTC"=w601, "Latitude"=w600, "Longitude"=w599, "Speed over ground"=w598, "Course over ground"=w597) -> (w602:T1)
      }
      frame "VTG" {
        w617 = T16 {"Heading_T"=0.0, "T"=0, "Heading_M"=0.0, "M"=0, "G_Speed_Knote"=0.0, "N"=0, "G_Speed_KPH"=0.0}  # 클러스터 2
        n253 = Type Cast(type=w617, x=w618) -> (*(type *) &x=w616:T16)
        n254 = Unbundle By Name(w616) -> ("Heading_T"=w613:dbl, "Heading_M"=w611:dbl, "G_Speed_KPH"=w607:dbl)
        "Heading_M" <- w611
        "KHP" <- w607
        n255 = expression code="x*1000"(w607) -> (w609:dbl)
        n256 = To Unsigned Word Integer(number=w609) -> (unsigned 16bit integer=→"GPS_KHP":u16)
        n257 = Not Equal To 0?(x=w613) -> (x != 0?=w612:bool)
        n258 = case shown="True" w612 {
          tunnel: w613 -> [_ w619]
          tunnel: [_ w619] -> w610
          frame False {
          }
          frame True {
          }
        }
        "Heading_T" <- w610
        n259 = Bundle By Name(cluster=w614, "Heading_T"=w610, "Heading_P"=w611) -> (w615:T1)
      }
    }
    "F9P GPS Data" <- w568
    n260 = Unbundle By Name(w568) -> ("Latitude"=w573:dbl, "Longitude"=w552:dbl)
    n261 = expression code="x*100"(w552) -> (w553:dbl)
    n262 = expression code="x*100000"(w573) -> (w554:dbl)
    n263 = To Unsigned Quad Integer(1:w553) -> (0:→"TCP_Long":u64)
    n264 = To Unsigned Quad Integer(1:w554) -> (0:→"TCP_Lat":u64)
    n265 = call "TM_trans (SubVI).vi"("long"=w552, "lat"=w573) -> ("Y(long)"=→"TM_Y(long)":dbl, "X(lat)"=→"TM_X(lat)":dbl)  [unwired: 1 in]
    n266 = local read "stop"() -> (w555:bool)
  }
  n267 = while {
    tunnel: w24 -> [w667]
    tunnel: w23 -> [w666]
    tunnel: [w661] -> w26
    tunnel: [w660] -> w25
    i -> [w658]
    stop <- w634 stop-if-true
    # "BMS"
    n268 = Quotient & Remainder(x=w658, y=20) -> (x-y*floor(x/y)=w655:i32)  [unwired: 1 out]
    n269 = case shown="0..9, Default" w655 {
      tunnel: [TRUE FALSE] -> w656
      frame 0..9, Default {
      }
      frame 10..19 {
      }
    }
    n270 = Wait Until Next ms Multiple(millisecond multiple=u32 100 ("타임아웃(ms) (-1)")) -> ()  [unwired: 1 out]
    n271 = flat-sequence {
      tunnel: [w687] -> w669
      tunnel: [w686] -> w668
      tunnel: w667 -> [w685]
      tunnel: w666 -> [w684]
      tunnel: w656 -> [w681]
      tunnel: w669 -> [w692]
      tunnel: w668 -> [w691]
      tunnel: [w692] -> w665
      tunnel: [w691] -> w664
      tunnel: w665 -> [w726]
      tunnel: w664 -> [w725]
      tunnel: [w724] -> w663
      tunnel: [w723] -> w662
      tunnel: [w696] -> w654
      tunnel: [w695] -> w640
      tunnel: [w694] -> w639
      tunnel: [w693] -> w638
      tunnel: w663 -> [w732]
      tunnel: w662 -> [w731]
      tunnel: [w732] -> w661
      tunnel: [w731] -> w660
      tunnel: w654 -> [w730]
      tunnel: [w730] -> w650
      tunnel: [w729] -> w637
      tunnel: w640 -> [w729]
      tunnel: [w728] -> w636
      tunnel: w639 -> [w728]
      tunnel: [w727] -> w635
      tunnel: w638 -> [w727]
      frame #0 {
        (unwired) "\u0001\u0003Ð2\u0000\u0003œÄ"
        (unwired) "\u0001\u0003Ð%\u0000\u0001­\u0001"
        n272 = case shown="False" w681 {
          tunnel: ["\u0001\u0003Ð2\u0000\u0003œÄ" "\u0001\u0003Ð%\u0000\u0001­\u0001"] -> w682
          frame False {
          }
          frame True {
          }
        }
        n273 = Concatenate Strings(w682, "\r\n") -> (w683:string)
        n274 = VISA Write(VISA resource name=w685, write buffer=w683, error in (no error)=w684) -> (VISA resource name out=w687:refnum<visa-resource-name>, error out=w686:errorcluster)  [unwired: 1 out]
      }
      frame #1 {
        n275 = Wait (ms)(milliseconds to wait=u32 10) -> ()  [unwired: 1 out]
      }
      frame #2 {
        n276 = VISA Read(VISA resource name=w726, byte count=u32 200, error in (no error)=w725) -> (VISA resource name out=w724:refnum<visa-resource-name>, read buffer=w715:string, error out=w723:errorcluster)  [unwired: 1 out]
        n277 = Match Pattern(string=w715, regular expression="\u0001\u0003\u0002", offset (0)=0 ("offset past match")) -> (after substring=w719:string)  [unwired: 3 out]
        n278 = Match Pattern(string=w715, regular expression="\u0001\u0003\u0006", offset (0)=0 ("offset past match")) -> (after substring=w718:string)  [unwired: 3 out]
        n279 = String To Byte Array(string=w719) -> (unsigned byte array=w712:u8[])
        n280 = String To Byte Array(string=w718) -> (unsigned byte array=w705:u8[])
        n281 = Index Array(array=w705, index #1=0, index #2=1, index #3=2, index #4=3, index #5=4, index #6=5) -> (element #1=w709:u8, element #2=w708:u8, element #3=w700:u8, element #4=w699:u8, element #5=w698:u8, element #6=w697:u8)
        n282 = Index Array(array=w712, index #1=0, index #2=1) -> (element #1=w710:u8, element #2=w711:u8)
        n283 = Join Numbers(hi=w709, lo=w708) -> ((hi.lo)=w695:u16)
        n284 = Join Numbers(hi=w700, lo=w699) -> ((hi.lo)=w694:u16)
        n285 = Join Numbers(hi=w710, lo=w711) -> ((hi.lo)=w696:u16)
        n286 = Join Numbers(hi=w698, lo=w697) -> ((hi.lo)=w693:u16)
      }
      frame #3 {
        n287 = Wait (ms)(milliseconds to wait=u32 10) -> ()  [unwired: 1 out]
      }
    }
    n288 = Not Equal To 0?(x=w650) -> (x != 0?=w651:bool)
    n289 = Not Equal To 0?(x=w637) -> (x != 0?=w649:bool)
    n290 = Not Equal To 0?(x=w635) -> (x != 0?=w643:bool)
    n291 = Not Equal To 0?(x=w636) -> (x != 0?=w644:bool)
    n292 = feedback #1(u16 0) -> (w646:u16)
    n293 = case shown="True" w644 {
      tunnel: w636 -> [_ w673]
      tunnel: [w672 w673] -> w622
      tunnel: w646 -> [w672 _]
      frame False {
      }
      frame True {
      }
    }
    n294 = feedback-in #1(w622) -> ()
    n295 = feedback #2(u16 0) -> (w653:u16)
    n296 = case shown="True" w651 {
      tunnel: w650 -> [_ w677]
      tunnel: [w676 w677] -> w632
      tunnel: w653 -> [w676 _]
      frame False {
      }
      frame True {
      }
    }
    n297 = feedback-in #2(w632) -> ()
    n298 = feedback #3(u16 0) -> (w647:u16)
    n299 = case shown="True" w649 {
      tunnel: w637 -> [_ w675]
      tunnel: [w674 w675] -> w627
      tunnel: w647 -> [w674 _]
      frame False {
      }
      frame True {
      }
    }
    n300 = feedback-in #3(w627) -> ()
    n301 = feedback #4(u16 0) -> (w641:u16)
    n302 = case shown="True" w643 {
      tunnel: w635 -> [_ w671]
      tunnel: [w670 w671] -> w621
      tunnel: w641 -> [w670 _]
      frame False {
      }
      frame True {
      }
    }
    n303 = feedback-in #4(w621) -> ()
    n304 = To Double Precision Float(number=w632) -> (double precision float=w631:dbl)
    n305 = To Double Precision Float(number=w622) -> (double precision float=w625:dbl)
    n306 = To Unsigned Byte Integer(number=w621) -> (unsigned 8bit integer=→"SOC":u8)
    n307 = To Double Precision Float(number=w627) -> (double precision float=w628:dbl)
    n308 = Multiply(x=w631, y=0.01) -> (x*y=→"Batt_Volt":dbl)
    n309 = Multiply(x=w625, y=0.01) -> (x*y=→"Discharge":dbl)
    n310 = Multiply(x=w628, y=0.1) -> (x*y=→"Charge":dbl)
    n311 = local read "stop"() -> (w634:bool)
  }
  n312 = TCP Open Connection(address="121.166.167.135" ("service name"), remote port or service name=w2, timeout ms (60000)=w3) -> (connection ID=w10:refnum<k5>, error out=w9:errorcluster)  [unwired: 2 in]
  n313 = while {
    tunnel: [w790] -> w19
    tunnel: [w791] -> w20
    tunnel: w10 -> [w807]
    tunnel: w9 -> [w806]
    i -> [w808]
    stop <- w809 stop-if-true
    (unwired) T17."little-endian" ("byte order (0:big-endian, network order)")
    # "TCP Robot_TX"
    n314 = local read "Robot_State"() -> (w763:u8)
    n315 = local read "Robot_Mode"() -> (w734:u8)
    n316 = local read "TCP_Long"() -> (w788:u64)
    n317 = local read "TCP_Lat"() -> (w787:u64)
    n318 = Wait Until Next ms Multiple(millisecond multiple=u32 500 ("ms 배수")) -> ()  [unwired: 1 out]
    n319 = local read "SOC"() -> (w792:u8)
    n320 = local read "IMU_Output"() -> (w744:T6)
    n321 = Flatten To String(anything=u16 11, byte order (0:big-endian, network order)=T17."little-endian") -> (data string=w794:string)  [unwired: 2 in, 2 out]
    n322 = Flatten To String(anything=u16 3000, byte order (0:big-endian, network order)=T17."little-endian") -> (data string=w800:string)  [unwired: 2 in, 2 out]
    n323 = Flatten To String(anything=w792, byte order (0:big-endian, network order)=T17."little-endian") -> (data string=w799:string)  [unwired: 2 in, 2 out]
    n324 = Flatten To String(anything=w763, byte order (0:big-endian, network order)=T17."little-endian") -> (data string=w798:string)  [unwired: 2 in, 2 out]
    n325 = Flatten To String(anything=w734, byte order (0:big-endian, network order)=T17."little-endian") -> (data string=w796:string)  [unwired: 2 in, 2 out]
    n326 = Flatten To String(anything=w787) -> (data string=w785:string)  [unwired: 3 in, 2 out]
    n327 = Flatten To String(anything=w788, byte order (0:big-endian, network order)=T17."little-endian") -> (data string=w784:string)  [unwired: 2 in, 2 out]
    n328 = Unbundle By Name(w744) -> ("Acc_X"=w762:dbl, "Acc_Y"=w761:dbl, "Acc_Z"=w760:dbl, "Gyro_X"=w759:dbl, "Gyro_Y"=w758:dbl, "Gyro_Z"=w757:dbl, "Roll"=w756:dbl, "Pitch"=w755:dbl, "Yaw"=w754:dbl)
    n329 = expression code="x*1000"(w762) -> (w753:dbl)
    n330 = expression code="x*1000"(w761) -> (w752:dbl)
    n331 = expression code="x*1000"(w760) -> (w751:dbl)
    n332 = expression code="x*100"(w759) -> (w750:dbl)
    n333 = expression code="x*100"(w758) -> (w749:dbl)
    n334 = expression code="x*100"(w757) -> (w748:dbl)
    n335 = expression code="x*100"(w756) -> (w747:dbl)
    n336 = expression code="x*100"(w755) -> (w746:dbl)
    n337 = expression code="x*100"(w754) -> (w745:dbl)
    n338 = To Word Integer(number=w748) -> (16bit integer=w738:i16)
    n339 = To Word Integer(number=w750) -> (16bit integer=w740:i16)
    n340 = To Word Integer(number=w749) -> (16bit integer=w739:i16)
    n341 = To Word Integer(number=w745) -> (16bit integer=w735:i16)
    n342 = To Word Integer(number=w747) -> (16bit integer=w737:i16)
    n343 = To Word Integer(number=w746) -> (16bit integer=w736:i16)
    n344 = To Word Integer(number=w753) -> (16bit integer=w743:i16)
    n345 = To Word Integer(number=w752) -> (16bit integer=w742:i16)
    n346 = To Word Integer(number=w751) -> (16bit integer=w741:i16)
    n347 = Flatten To String(anything=w738, byte order (0:big-endian, network order)=T17."little-endian") -> (data string=w773:string)  [unwired: 2 in, 2 out]
    n348 = Flatten To String(anything=w739, byte order (0:big-endian, network order)=T17."little-endian") -> (data string=w774:string)  [unwired: 2 in, 2 out]
    n349 = Flatten To String(anything=w740, byte order (0:big-endian, network order)=T17."little-endian") -> (data string=w775:string)  [unwired: 2 in, 2 out]
    n350 = Flatten To String(anything=w741, byte order (0:big-endian, network order)=T17."little-endian") -> (data string=w778:string)  [unwired: 2 in, 2 out]
    n351 = Flatten To String(anything=w742, byte order (0:big-endian, network order)=T17."little-endian") -> (data string=w780:string)  [unwired: 2 in, 2 out]
    n352 = Flatten To String(anything=w743, byte order (0:big-endian, network order)=T17."little-endian") -> (data string=w783:string)  [unwired: 2 in, 2 out]
    n353 = local read "GPS_KHP"() -> (w766:u16)
    n354 = Flatten To String(anything=w766, byte order (0:big-endian, network order)=T17."little-endian") -> (data string=w764:string)  [unwired: 2 in, 2 out]
    n355 = Flatten To String(anything=w735, byte order (0:big-endian, network order)=T17."little-endian") -> (data string=w767:string)  [unwired: 2 in, 2 out]
    n356 = Flatten To String(anything=w736, byte order (0:big-endian, network order)=T17."little-endian") -> (data string=w768:string)  [unwired: 2 in, 2 out]
    n357 = Flatten To String(anything=w737, byte order (0:big-endian, network order)=T17."little-endian") -> (data string=w769:string)  [unwired: 2 in, 2 out]
    n358 = local read "stop"() -> (w809:bool)
    n359 = Concatenate Strings(w794, w800, w799, w798, w796, w785, w784, w783, w780, w778, w775, w774, w773, w769, w768, w767, w764) -> (w793:string)
    n360 = TCP Write(connection ID=w807, data in=w793, error in (no error)=w806) -> (connection ID out=w791:refnum<k5>, error out=w790:errorcluster)  [unwired: 2 out]
    "bytes written" <- w808
  }
  n361 = while {
    tunnel: w10 -> [w815]
    tunnel: w9 -> [w814]
    tunnel: [w813] -> w8
    tunnel: [w812] -> w7
    stop <- w811 stop-if-true
    # "TCP RX"
    n362 = TCP Read(connection ID=w815, bytes to read=5, error in (no error)=w814) -> (connection ID out=w813:refnum<k5>, data out=w816:string, error out=w812:errorcluster)  [unwired: 2 in]
    n363 = Wait Until Next ms Multiple(millisecond multiple=u32 500 ("ms 배수")) -> ()  [unwired: 1 out]
    n364 = String To Byte Array(string=w816) -> (unsigned byte array=w817:u8[])
    n365 = Index Array(array=w817, index #1=3, index #2=2) -> (element #1=w821:u8, element #2=w822:u8)
    n366 = Join Numbers(hi=w821, lo=w822) -> ((hi.lo)=w820:u16)
    n367 = Equal?(x=u16 3001, y=w820) -> (x = y?=w818:bool)
    n368 = case shown="True" w818 {
      tunnel: w817 -> [_ w829]
      frame False {
      }
      frame True {
        n369 = Index Array(array=w829, index=4) -> (element=→"Go&Stop_CMD":u8)
      }
    }
    n370 = local read "stop"() -> (w811:bool)
  }
  n371 = VISA Close(VISA resource name=w46, error in (no error)=w45) -> (error out=w41:errorcluster)
  n372 = call <vilib>:"Clear Errors.vi"("error in (no error)"=w41) -> ()  [unwired: 5 in, 2 out]
  n373 = TCP Close Connection(connection ID=w8, error in (no error)=w7) -> (error out=w6:errorcluster)  [unwired: 2 out]
  n374 = TCP Close Connection(connection ID=w20, error in (no error)=w19) -> (error out=w5:errorcluster)  [unwired: 2 out]
  n375 = Merge Errors(w6, w5) -> (w4:errorcluster)
  n376 = call <vilib>:"Simple Error Handler.vi"("error in (no error)"=w4) -> ()  [unwired: 4 in, 5 out]
  n377 = VISA Close(VISA resource name=w26, error in (no error)=w25) -> (error out=w22:errorcluster)
  n378 = call <vilib>:"Clear Errors.vi"("error in (no error)"=w22) -> ()  [unwired: 5 in, 2 out]
